vi "MAIN_MEMS_NL.vi"() -> ()   [LabVIEW 2017]
uses:
  <vilib>/Utility/file.llb/Write Delimited Spreadsheet (DBL).vi
  Agilent 33220A/Agilent 33XXX Series.lvlib
  Agilent 2000 3000 X-Series/Agilent 2000 3000 X-Series.lvlib
panel:
  out "Current OSC":ext
  out "Current Vdc":ext
  in  "Variable_Tab":enum32{"OSC"}(tab)
  in  "Vt [V]":ext
  in  "Start Osc [mV]":ext=500.0
  in  "Stop Osc [mV]":ext=500.0
  in  "Step Osc [mV]":ext=10.0
  out "Burst Phase":dbl=100.0 caption="Burst Phase [deg]"
  in  "Burst period":ext=12.0 caption="Burst period [ms]"
  in  "N_acquisition":i32=100
  in  "Start Vdc [V]":ext=7.0
  in  "Stop Vdc [V]":ext=7.0
  in  "Step Vdc [V]":ext=0.25
  in  "Save":bool caption="SAVE?"
  in  "Start Freq [Hz]":ext=418000.0
  in  "Stop Freq [Hz]":ext=418000.0
  in  "Step Freq [Hz]":ext=500.0
  in  "mV/div [CH1]":ext=17.0
  in  "mV/div [CH2]":dbl=660.0 format="%#_13g"
  in  "Vertical Offset CH2":dbl=1.5 caption="Vertical Offset CH2 [V]" format="%#_13g"
  in  "Vertical Offset CH1":dbl=0.013 caption="Vertical Offset CH1 [V]"
  in  "string":string="Zsign_1MOhm_ZOscill_1MOhm_D4_Rf_500kOhm_G_10"
  out "Averaged":cluster{dbl[], "Y":dbl[]}[](graph)
  in  "Path":path=path "C:/Users/MEMSlab4/Desktop/Progetti_ES2M/Avanzi_Corazzina/Misure"
  # "Pk-Pk"
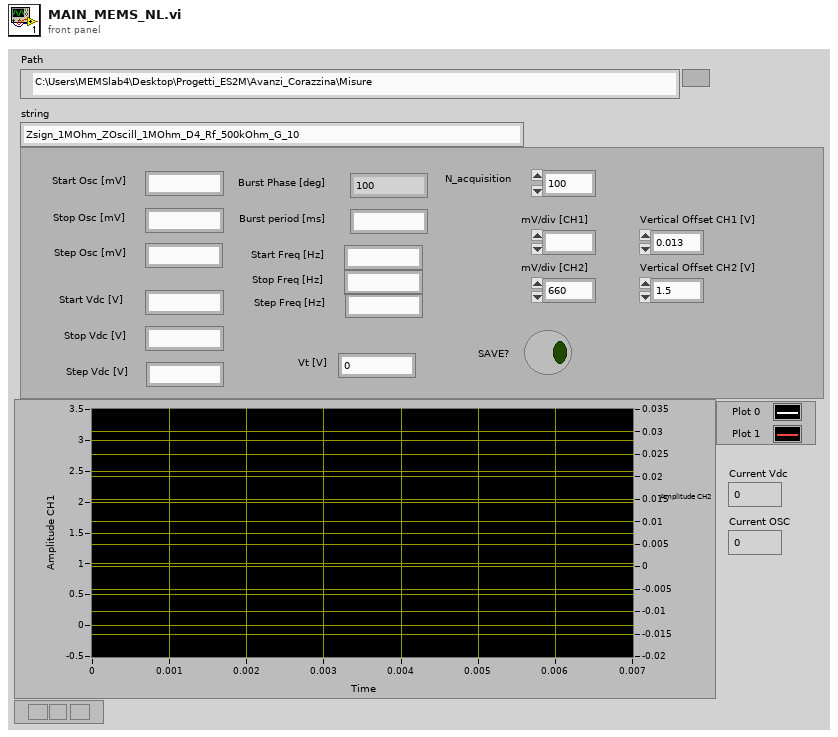
[diagram p1: front panel]
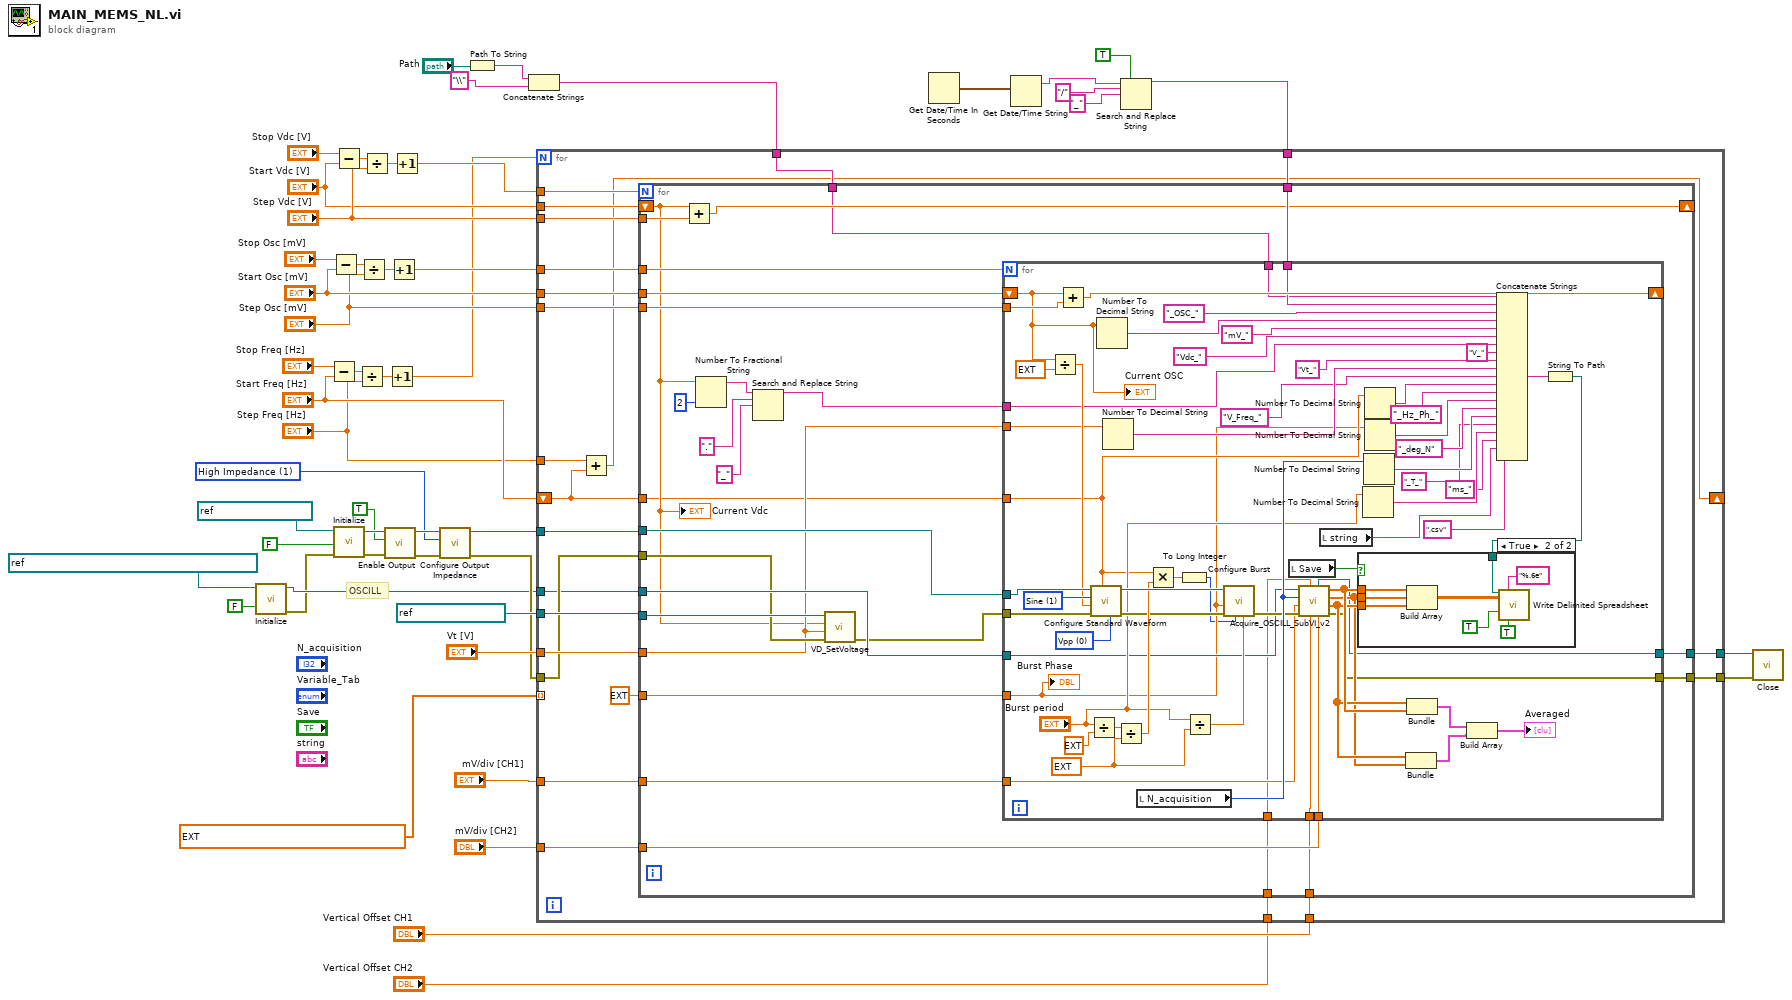
[diagram p0: block diagram]
diagram:
  w19 = u16 1 items=["50 Ohms", "High Impedance", "User Defined"] ("Impedance (0: 50 Ohms)")
  # "OSCILL"
  n1 = call "Initialize.vi"("Reset (True)"=FALSE, "VISA resource name"=refnum<visa-resource-name> "USB0::0x0957::0x17A8::MY52100688::INSTR" ("VISA Refnum in")) -> ("error out"=w15:errorcluster, "VISA resource name out"=w16:refnum<visa-resource-name>)  [unwired: 3 in, 5 out]
  n2 = Subtract(x="Stop Freq [Hz]", y="Start Freq [Hz]") -> (x-y=w10:ext)
  n3 = Subtract(x="Stop Osc [mV]", y="Start Osc [mV]") -> (x-y=w36:ext)
  n4 = Subtract(x="Stop Vdc [V]", y="Start Vdc [V]") -> (x-y=w28:ext)
  n5 = call "Initialize.vi"("error in (no error)"=w15, "Reset (True)"=FALSE, "VISA resource name"=refnum<visa-resource-name> "GPIB0::10::INSTR") -> ("error out"=w48:errorcluster, "VISA resource name out"=w49:refnum<visa-resource-name>)  [unwired: 7 in]
  n6 = Divide(x=w10, y="Step Freq [Hz]") -> (x/y=w9:ext)
  n7 = Divide(x=w36, y="Step Osc [mV]") -> (x/y=w37:ext)
  n8 = Divide(x=w28, y="Step Vdc [V]") -> (x/y=w27:ext)
  n9 = call "Enable Output.vi"("error in (no error)"=w48, "Enable Output  (T: Enable)"=TRUE, "VISA resource name"=w49) -> ("error out"=w22:errorcluster, "VISA resource name out"=w23:refnum<visa-resource-name>)  [unwired: 7 in]
  n10 = Increment(x=w9) -> (x+1=w8:ext)
  n11 = Increment(x=w37) -> (x+1=w34:ext)
  n12 = Increment(x=w27) -> (x+1=w26:ext)
  n13 = call "Configure Output Impedance.vi"("error in (no error)"=w22, "Impedance (0: 50 Ohms)"=w19, "VISA resource name"=w23) -> ("error out"=w21:errorcluster, "VISA resource name out"=w20:refnum<visa-resource-name>)  [unwired: 7 in]
  n14 = Path To String(path="Path") -> (string=w45:string)
  n15 = Concatenate Strings(w45, "\\" ("string")) -> (w30:string)
  n16 = Get Date/Time In Seconds() -> (seconds since 1Jan1904=w43:timestamp)
  n17 = Get Date/Time String(seconds (now)=w43) -> (date string=w40:string)  [unwired: 2 in, 1 out]
  n18 = Search and Replace String(replace all?=TRUE ("replace all? (F)"), input string=w40, search string="/", replace string="_" ("replace string (\"\")")) -> (result string=w12:string)  [unwired: 4 in, 3 out]
  n19 = for {
    N: w8 -> [_]
    tunnel: w34 -> [w73]
    tunnel: "Start Osc [mV]" -> [w72]
    tunnel: "Step Osc [mV]" -> [w71]
    tunnel: "Vt [V]" -> [w70]
    tunnel: w30 -> [w69]
    tunnel: w26 -> [w68]
    tunnel: "Step Vdc [V]" -> [w67]
    tunnel: "Start Vdc [V]" -> [w66]
    tunnel: w20 -> [w64]
    tunnel: w16 -> [w63]
    tunnel: w12 -> [w60]
    tunnel: refnum<visa-resource-name> "GPIB0::5::INSTR" ("VISA Refnum in") -> [w74]
    tunnel: [w62] -> w14
    tunnel: w21 -> [w65]
    tunnel: [w61] -> w13
    shift-right: [w57] -> _
    shift-left: "Start Freq [Hz]" -> [w59]
    tunnel: "Step Freq [Hz]" -> [w58]
    tunnel: "mV/div [CH1]" -> [w56]
    tunnel: ext[] [104.0, 97.0, 93.0, 96.0, 97.0, 95.0, 95.0] ("Vt [V] 2") -> [_] mode=indexing
    tunnel: "mV/div [CH2]" -> [w54]
    tunnel: "Vertical Offset CH1" -> [w53]
    tunnel: "Vertical Offset CH2" -> [w52]
    n20 = Add(x=w58, y=w59) -> (x+y=w57:ext)
    n21 = for {
      N: w68 -> [_]
      tunnel: w64 -> [w101]
      tunnel: w63 -> [w100]
      tunnel: w74 -> [w99]
      tunnel: w65 -> [w98]
      tunnel: w73 -> [w97]
      tunnel: w72 -> [w96]
      tunnel: w71 -> [w95]
      tunnel: w70 -> [w93]
      tunnel: w60 -> [w92]
      tunnel: w69 -> [w81]
      tunnel: w67 -> [w91]
      shift-right: [w90] -> _
      shift-left: w66 -> [w84]
      tunnel: w59 -> [w80]
      tunnel: [w83] -> w62
      tunnel: [w82] -> w61
      tunnel: w56 -> [w79]
      tunnel: ext 93.0 ("Vt [V] 2") -> [w78]
      tunnel: w54 -> [w77]
      tunnel: w53 -> [w76]
      tunnel: w52 -> [w75]
      n22 = Add(x=w84, y=w91) -> (x+y=w90:ext)
      n23 = Number To Fractional String(number=w84, precision (6)=i16 2) -> (F-format string=w85:string)  [unwired: 2 in]
      n24 = Search and Replace String(input string=w85, search string=".", replace string="_" ("replace string (\"\")")) -> (result string=w87:string)  [unwired: 5 in, 3 out]
      n25 = call "VD_SetVoltage.vi"("error in"=w98, "Vout2"=w93, "Vout1"=w84, "VISA VD_Supply"=w99) -> ("error out"=w94:errorcluster)  [unwired: 6 in, 1 out]
      n26 = for {
        N: w97 -> [_]
        tunnel: w101 -> [w162]
        shift-right: [w160] -> _
        shift-left: w96 -> [w116]
        tunnel: w95 -> [w147]
        tunnel: w100 -> [w111]
        tunnel: w94 -> [w144]
        tunnel: w93 -> [w141]
        tunnel: w87 -> [w117]
        tunnel: w81 -> [w109]
        tunnel: w92 -> [w110]
        tunnel: w80 -> [w115]
        tunnel: [w114] -> w83
        tunnel: [w112] -> w82
        tunnel: w79 -> [w108]
        tunnel: w78 -> [w107]
        tunnel: w77 -> [w105]
        tunnel: w76 -> [w103]
        tunnel: w75 -> [w102]
        w125 = ext 1000.0 ("y")
        w157 = u16 0 items=["Vpp", "Vrms", "dB"] ("Unit (0: Vpp)")
        w161 = u16 1 items=["DC", "Sine", "Square", "Triangle", "Ramp", "Pulse", "Noise", "Sinc", "Negative Ramp", "Exponential Rise", "Exponential Fall", "Cardiac"] ("Waveform Function (1: Sine)")
        n27 = Divide(x=w116, y=ext 1000.0) -> (x/y=w158:ext)
        n28 = Add(x=w116, y=w147) -> (x+y=w160:ext)
        n29 = Divide(x="Burst period", y=ext 2.0) -> (x/y=w153:ext)
        n30 = call "Configure Standard Waveform.vi"("Unit (0: Vpp)"=w157, "Frequency (1000 Hz)"=w115, "error in (no error)"=w144, "Amplitude (1)"=w158, "Waveform Function (1: Sine)"=w161, "VISA resource name"=w162) -> ("error out"=w151:errorcluster, "VISA resource name out"=w156:refnum<visa-resource-name>)  [unwired: 4 in]
        n31 = Number To Decimal String(number=w116) -> (decimal integer string=w146:string)  [unwired: 1 in]
        n32 = Number To Decimal String(number=w141) -> (decimal integer string=w140:string)  [unwired: 1 in]
        n33 = Divide(x=w153, y=w125) -> (x/y=w152:ext)
        n34 = local read "N_acquisition"() -> (w133:i32)
        n35 = Multiply(x=w115, y=w152) -> (x*y=w155:ext)
        n36 = To Long Integer(number=w155) -> (32bit integer=w104:i32)
        n37 = Divide(x="Burst period", y=w125) -> (x/y=w124:ext)
        n38 = call "Configure Burst.vi"("Burst Period (1 s)"=w124, "Burst Count (1)"=w104, "error in (no error)"=w151, "Burst Phase (0 deg)"=w107, "VISA resource name"=w156) -> ("error out"=w113:errorcluster)  [unwired: 5 in, 1 out]
        n39 = local read "Save"() -> (w150:bool)
        n40 = call "Acquire_OSCILL_SubVI_v2.vi"("mV/div [CH2]"=w105, "Vertical Offset CH1"=w103, "Vertical Offset CH2"=w102, "error in (no error)"=w113, "mV/div [CH1]"=w108, "N_acquisition"=w133, "VISA resource name"=w111) -> ("error out"=w112:errorcluster, "Time"=w127:dbl[], "CH2_averaged"=w126:dbl[], "CH1_averaged"=w128:dbl[], "VISA resource name out"=w114:refnum<visa-resource-name>)
        n41 = local read "string"() -> (w119:string)
        n42 = Number To Decimal String(number="Burst period") -> (decimal integer string=w121:string)  [unwired: 1 in]
        n43 = Number To Decimal String(number=w133) -> (decimal integer string=w134:string)  [unwired: 1 in]
        n44 = Number To Decimal String(number=w115) -> (decimal integer string=w138:string)  [unwired: 1 in]
        n45 = Number To Decimal String(number=w107) -> (decimal integer string=w136:string)  [unwired: 1 in]
        n46 = Bundle("Time"=w127, "CH2_averaged"=w126) -> (w130:cluster{"Time":dbl[], "CH2_averaged":dbl[]})  [unwired: 1 in]
        n47 = Bundle("Time"=w127, "CH1_averaged"=w128) -> (w131:cluster{"Time":dbl[], "CH1_averaged":dbl[]})  [unwired: 1 in]
        n48 = Build Array(w131, w130) -> (→"Averaged":cluster{"Time":dbl[], "CH2_averaged":dbl[]}[])
        n49 = Concatenate Strings(w109, w110, "_OSC_" ("string"), w146, "mV_" ("string"), "Vdc_" ("string"), w117, "V_" ("string"), "Vt_" ("string"), w140, "V_Freq_" ("string"), w138, "_Hz_Ph_" ("string"), w136, "_deg_N" ("string"), w134, "_T_" ("string"), w121, "ms_" ("string"), w119, ".csv" ("string")) -> (w149:string)
        n50 = String To Path(string=w149) -> (path=w132:path)
        n51 = case shown="True" w150 {
          tunnel: w128 -> [_ w168]
          tunnel: w126 -> [_ w167]
          tunnel: w127 -> [_ w166]
          tunnel: w132 -> [_ w164]
          frame False {
          }
          frame True {
            n52 = Build Array(w168, w167, w166) -> (w165:dbl[][])
            n53 = call-poly <vilib>:"Write Delimited Spreadsheet.vi"("file path (dialog if empty)"=w164, "format (%.3f)"="%.6e", "2D data"=w165, "append to file? (new file:F)"=TRUE, "transpose? (no:F)"=TRUE) -> ()  [unwired: 9 in, 2 out]
          }
        }
        "Burst Phase" <- w107
        "Current OSC" <- w116
      }
      "Current Vdc" <- w84
    }
  }
  n54 = call "Close.vi"("error in (no error)"=w13, "VISA resource name"=w14) -> ()  [unwired: 10 out]
